vi "GetOutputShapeDimCount.vi"(8 "error in (no error)":errorcluster, 10 "outputIndex":i32, 11 "session id in":i32) -> (0 "error out":errorcluster, 2 "OutputShapeDimCount":i32, 3 "session id out":i32)   [LabVIEW 2017, in "libonnx_wrapper.lvlib"]
doc: "/**\n * @brief Получить количество размерностей выходного тензора\n * \n * Возвращает ранг тензора (число измерений). Например:\n * - Вектор [10] имеет 1 размерность\n * - Матрица [1, 10] имеет 2 размерности\n * - Изображение [1, 3, 224, 224] имеет 4 размерности\n * \n * @param sessionId [IN] ID сессии\n * @param outputIndex [IN] Индекс входа (0-based)\n * \n * @return int32: Количество размерностей (1, 2, 3, 4, ...)\n * @return int32: 0 если сессия не найдена или индекс неверен\n */\nint GetOutputShapeDimCount(int sessionId, int outputIndex);"
uses:
  libonnx_wrapper.lvlib
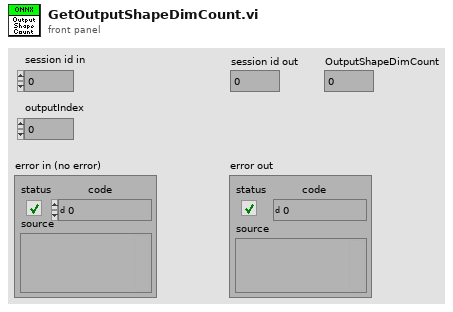
[diagram p1: front panel]
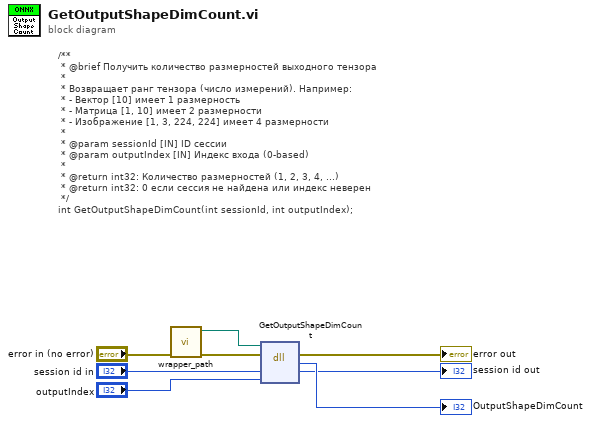
[diagram p0: block diagram]
diagram:
  # "/**\n * @brief Получить количество размерностей выходного тензора\n * \n * Возвращает ранг тензора (число измерений). Например:\n * - Вектор [10] имеет 1 размерность\n * - Матрица [1, 10] имеет 2 размерности\n * - Изображение [1, 3, 224, 224] имеет 4 размерности\n * \n * @param sessionId [IN] ID сессии\n * @param outputIndex [IN] Индекс входа (0-based)\n * \n * @return int32: Количество размерностей (1, 2, 3, 4, ...)\n * @return int32: 0 если сессия не найдена или индекс неверен\n */\nint GetOutputShapeDimCount(int sessionId, int outputIndex);"
  n1 = call "wrapper_path.vi"("error in (no error)"="error in (no error)") -> ("error out"=w2:errorcluster, "wrapper path"=w5:path)  [unwired: 9 in]
  n2 = dll-call lib="home/ivan/LabVIEWData/ONNX/Test/libonnx_wrapper/unix64/libonnx_wrapper.so" fn="GetOutputShapeDimCount"(path in=w5, error in=w2, "sessionId"="session id in", "inputIndex"="outputIndex") -> (error out=→"error out":errorcluster, "OutputShapeDimCount"=→"OutputShapeDimCount":i32, "sessionId"=→"session id out":i32)  [unwired: 2 in, 1 out]
